vi "Dequeue Job.vi"(8 "error in (no error)":errorcluster, 9 "timeout in ms (-1)":i32=-1, 11 "Mock Job Handler In":refnum<class "Mock Job Handler.lvclass">) -> (0 "error out":errorcluster, 1 "timed out?":bool, 2 "element":refnum<class>, 3 "Mock Job Handler Out":refnum<class "Mock Job Handler.lvclass">)   [LabVIEW 2020, in "Mock Job Handler.lvclass"]
uses:
  Mock Job Handler.lvclass
  Mock Job Handler.lvclass/Mock Job Handler.ctl
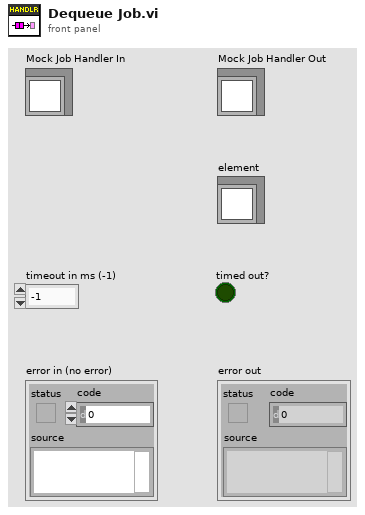
[diagram p1: front panel]
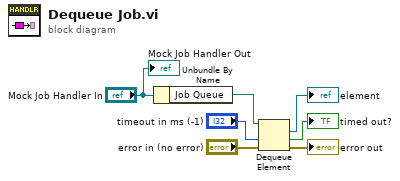
[diagram p0: block diagram]
diagram:
  n1 = Unbundle By Name("Mock Job Handler In") -> ("Job Queue"=w4:refnum<queue>)
  n2 = Dequeue Element(queue=w4, timeout in ms (-1)="timeout in ms (-1)", error in (no error)="error in (no error)") -> (element=→"element":refnum<class>, timed out?=→"timed out?":bool, error out=→"error out":errorcluster)  [unwired: 1 out]
  "Mock Job Handler Out" <- "Mock Job Handler In"
